vi "Get Text Rect with Pixel Font.vi"(8 "string":string="Hello", 10 "origin":cluster{"x":i16, "y":i16}) -> (2 "Rectangle out":T1)   [LabVIEW 2021, in "Picture Pixel Fonts.lvlib"]
uses:
  <vilib>/LabVIEW Icon API/Pixel Fonts/Picture Pixel Fonts.lvlib
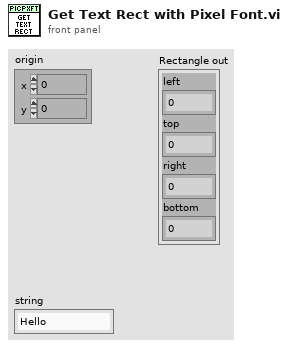
[diagram p1: front panel]
types:
  T1 = cluster{"left":i16, "top":i16, "right":i16, "bottom":i16}
  T2 = typedef "imagedata.ctl" = cluster{"image type":i32, "image depth":i32, "image":u8[], "mask":u8[], "colors":u32[], "Rectangle":cluster{"left":i16, "top":i16, "right":i16, "bottom":i16}}
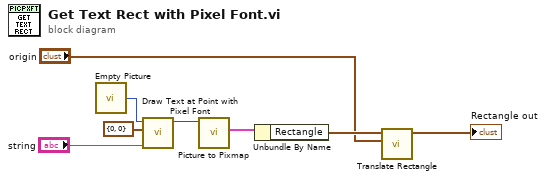
[diagram p0: block diagram]
diagram:
  n1 = call "Empty Picture"() -> ("empty picture"=w7:picture)
  n2 = call <vilib>:"Draw Text at Point with Pixel Font.vi"("string"="string", "origin"=cluster{"x":i16, "y":i16} {"x"=0, "y"=0}, "picture"=w7) -> ("picture out"=w5:picture)  [unwired: 8 in]
  n3 = call <vilib>:"Picture to Pixmap.vi"("picture"=w5) -> ("image data"=w4:T2)  [unwired: 9 in, 1 out]
  n4 = Unbundle By Name(w4) -> ("Rectangle"=w3:T1)
  n5 = call <vilib>:"Translate Rectangle.vi"("offset"="origin", "Rectangle in"=w3) -> ("Rectangle out"=→"Rectangle out":T1)  [unwired: 9 in]
